vi "Map - Get.vi"(8 "error in (no error)":errorcluster, 10 "Key":string, 11 "Map In":variant) -> (0 "error out":errorcluster, 1 "Found?":bool, 2 "Value":variant, 3 "Map Out":variant)   [LabVIEW 2024]
doc: "Gets value from <b>Map</b>."
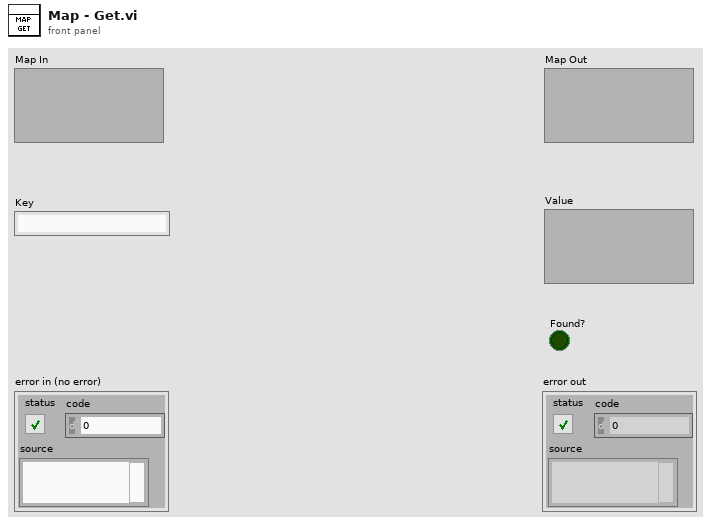
[diagram p1: front panel]
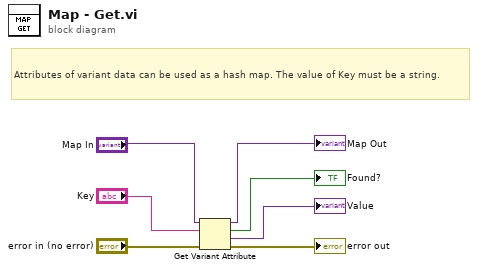
[diagram p0: block diagram]
diagram:
  # "Attributes of variant data can be used as a hash map. The value of Key must be a string."
  n1 = Get Variant Attribute(Variant="Map In", name="Key", error in="error in (no error)") -> (duplicate Variant=→"Map Out":variant, found=→"Found?":bool, value=→"Value":variant, error out=→"error out":errorcluster)  [unwired: 1 in]
